vi "Weibull PDF.vi"(9 "b":dbl=3.0, 10 "a":dbl=1.0, 11 "x":dbl=1.0) -> (0 "error":i32, 3 "pdf(x)":dbl=1.103638323514327)   [LabVIEW 2020, in "NI_Gmath.lvlib"]
doc: "Computes the continuous probability density function (PDF) of various distributions. You must manually select the polymorphic instance to use."
uses:
  NI_Gmath.lvlib
  st_error_code.ctl
panel:
  # "Weibull PDF"
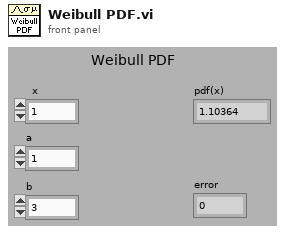
[diagram p1: front panel]
types:
  T1 = typedef "NI_Gmath.lvlib/st_error_code.ctl" = i32
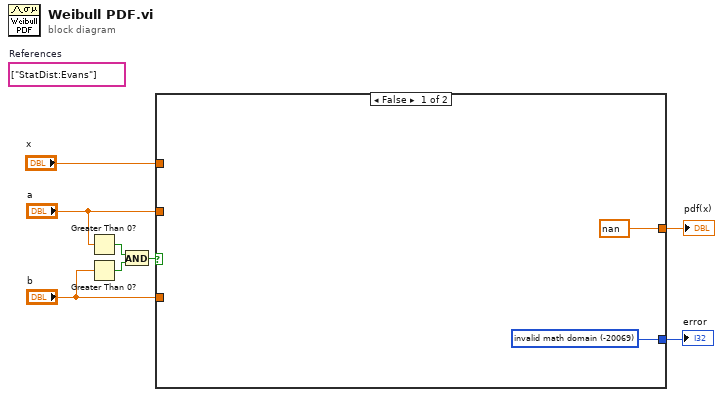
[diagram p0: block diagram]
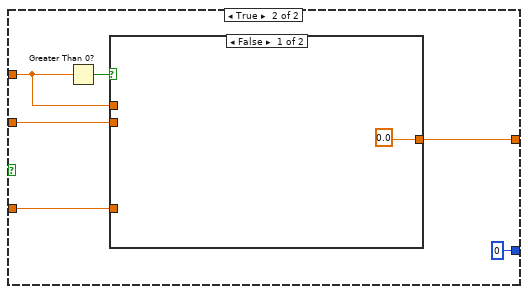
[diagram p2: hidden frame]
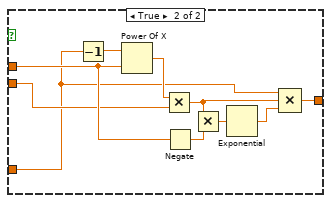
[diagram p3: hidden frame]
diagram:
  (unwired) string[] ["StatDist:Evans"]  # References
  n1 = Greater Than 0?(x="a") -> (x > 0?=w1:bool)
  n2 = Greater Than 0?(x="b") -> (x > 0?=w2:bool)
  n3 = And(x=w1, y=w2) -> (x .and. y?=w3:bool)
  n4 = case shown="False" w3 {
    tunnel: "b" -> [_ w13]
    tunnel: [w9 0 ("invalid math domain")] -> w8
    tunnel: [nan w15] -> w7
    tunnel: "x" -> [_ w11]
    tunnel: "a" -> [_ w14]
    frame False {
      w9 = T1 -20069 items=["invalid math domain"=-20069, "Fourier interpolation size m >= n"=-20070, "empty array"=-20003] ("stat interp error code")
    }
    frame True {
      n5 = Greater Than 0?(x=w11) -> (x > 0?=w12:bool)
      n6 = case shown="False" w12 {
        tunnel: [0.0 w21] -> w15
        tunnel: w11 -> [_ w25]
        tunnel: w14 -> [_ w19]
        tunnel: w13 -> [_ w18]
        frame False {
        }
        frame True {
          n7 = Decrement(x=w18) -> (x-1=w27:dbl)
          n8 = Power Of X(1:w25, 2:w27) -> (0:w26:dbl)
          n9 = Multiply(x=w26, y=w19) -> (x*y=w20:dbl)
          n10 = Negate(x=w25) -> (-x=w24:dbl)
          n11 = Multiply(x=w20, y=w24) -> (x*y=w23:dbl)
          n12 = Exponential(1:w23) -> (0:w22:dbl)
          n13 = Compound Arithmetic op=MULTIPLY(w18, w20, w22) -> (w21:dbl)
        }
      }
    }
  }
  "pdf(x)" <- w7
  "error" <- w8
